vi "getParameters.vi"(11 "StartCommand in":refnum<class "StartCommand.lvclass">) -> (2 "Parameters":T1, 3 "StartCommand out":refnum<class "StartCommand.lvclass">)   [LabVIEW 2016, in "StartCommand.lvclass"]
uses:
  StartCommand.lvclass
  DataTypes/Topics/CommandStart.ctl
  DataTypes/Topics/Parts/CommandId.ctl
  StartCommand.lvclass/StartCommand.ctl
  DataTypes/Topics/M1M3SupportTopics.lvlib
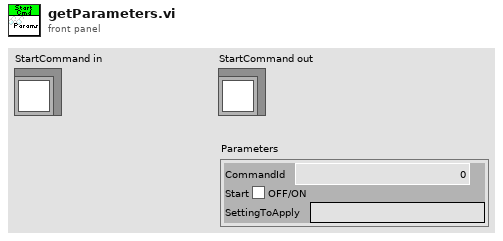
[diagram p1: front panel]
types:
  T1 = typedef "M1M3SupportTopics.lvlib/CommandStart.ctl" = cluster{"CommandId":T2, "Start":bool, "SettingToApply":string}
  T2 = typedef "M1M3SupportTopics.lvlib/CommandId.ctl" = i32
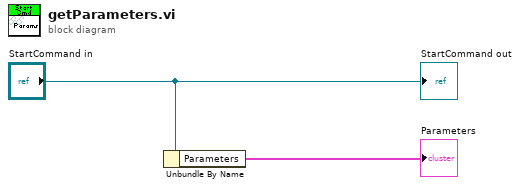
[diagram p0: block diagram]
diagram:
  n1 = Unbundle By Name("StartCommand in") -> ("Parameters"=→"Parameters":T1)
  "StartCommand out" <- "StartCommand in"
